vi "select device register.vi"(2 "Camera registers (T) / All Registers (F)":bool, 7 "Ok Button":string) -> (4 "Selected Register":T1, 8 "Register Selected":bool)   [LabVIEW 2010]
panel:
  out "Register Address:":dbl
  out "Raw Register Name:":string
  in  "Cancel":bool
  in  "Select":bool
  out "Pin name on the board:":string
  in  "Register:":u16(ring) items=["Camera on Digital 0 - Bit 0", "Camera on Digital 1 - Bit 0"]
  in  "Device:":u16(ring) items=["Common on all devices", "Behavior", "Camera Controller", "Multi Pwm", "Synchronizer", "Wear"]
  in  "read 5":bool
  in  "read 4":bool
  in  "read":bool
  in  "read 6":bool
  in  "read 7":bool
  in  "read 8":bool
  in  "read 3":bool
  in  "device":refnum<visa-resource-name>="COM5"
  # "Options:"
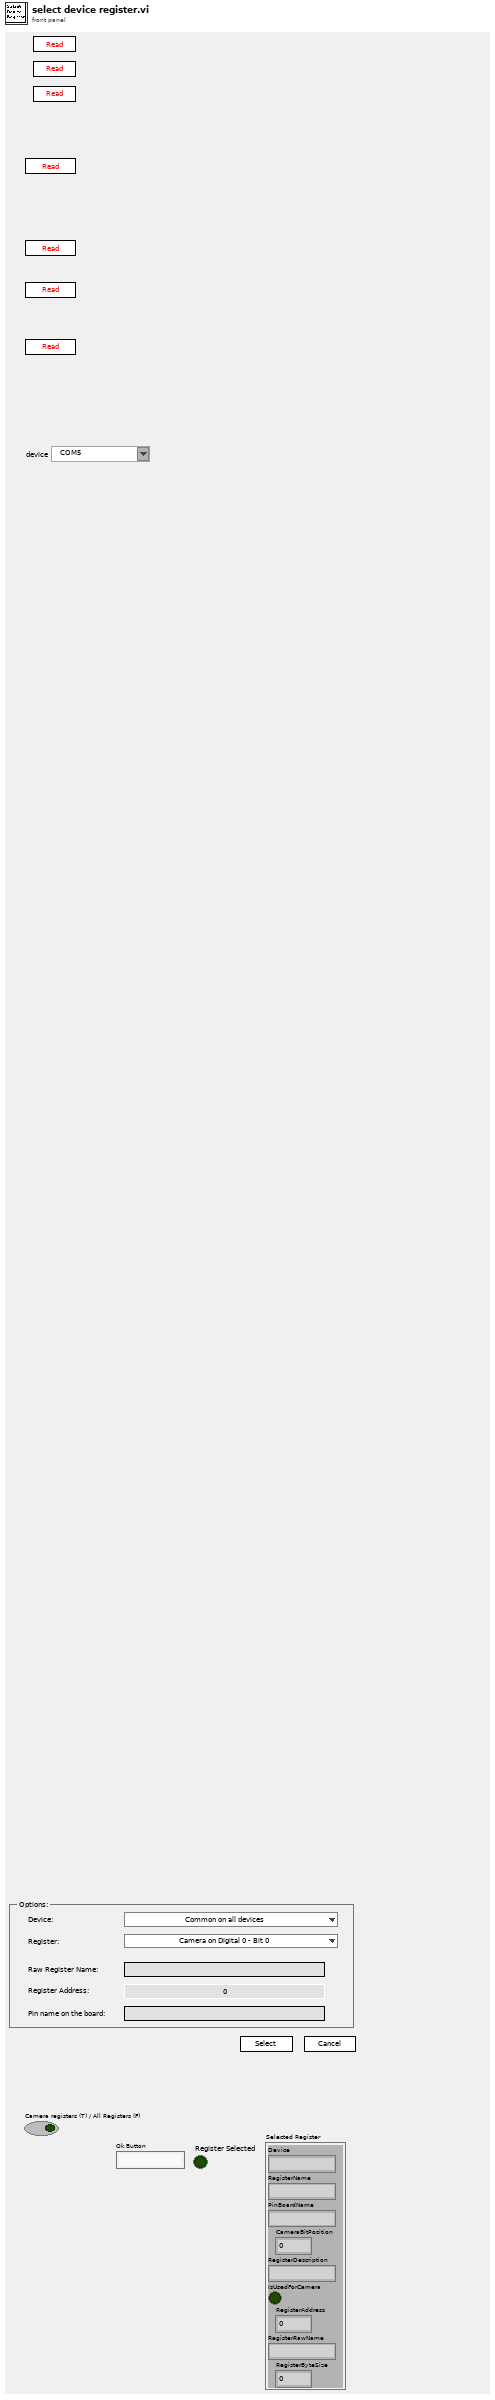
[diagram p1: front panel]
types:
  T1 = cluster{"Device":string, "RegisterName":string, "PinBoardName":string, "CameraBitPosition":i32, "RegisterDescription":string, "IsUsedForCamera":bool, "RegisterAddress":i32, "RegisterRawName":string, "RegisterByteSize":i32}
  T2 = cluster{"Device":string, "RegisterName":string, "PinBoardName":string, "CameraBitPosition":i32, "RegisterDescription":string, "IsUsedForCamera":bool, "RegisterAddress":i32, "RegisterRawName":string, "RegisterByteSize":i32}[][]
  T3 = cluster{"Device":string, "RegisterName":string, "PinBoardName":string, "CameraBitPosition":i32, "RegisterDescription":string, "IsUsedForCamera":bool, "RegisterAddress":i32, "RegisterRawName":string, "RegisterByteSize":i32}[]
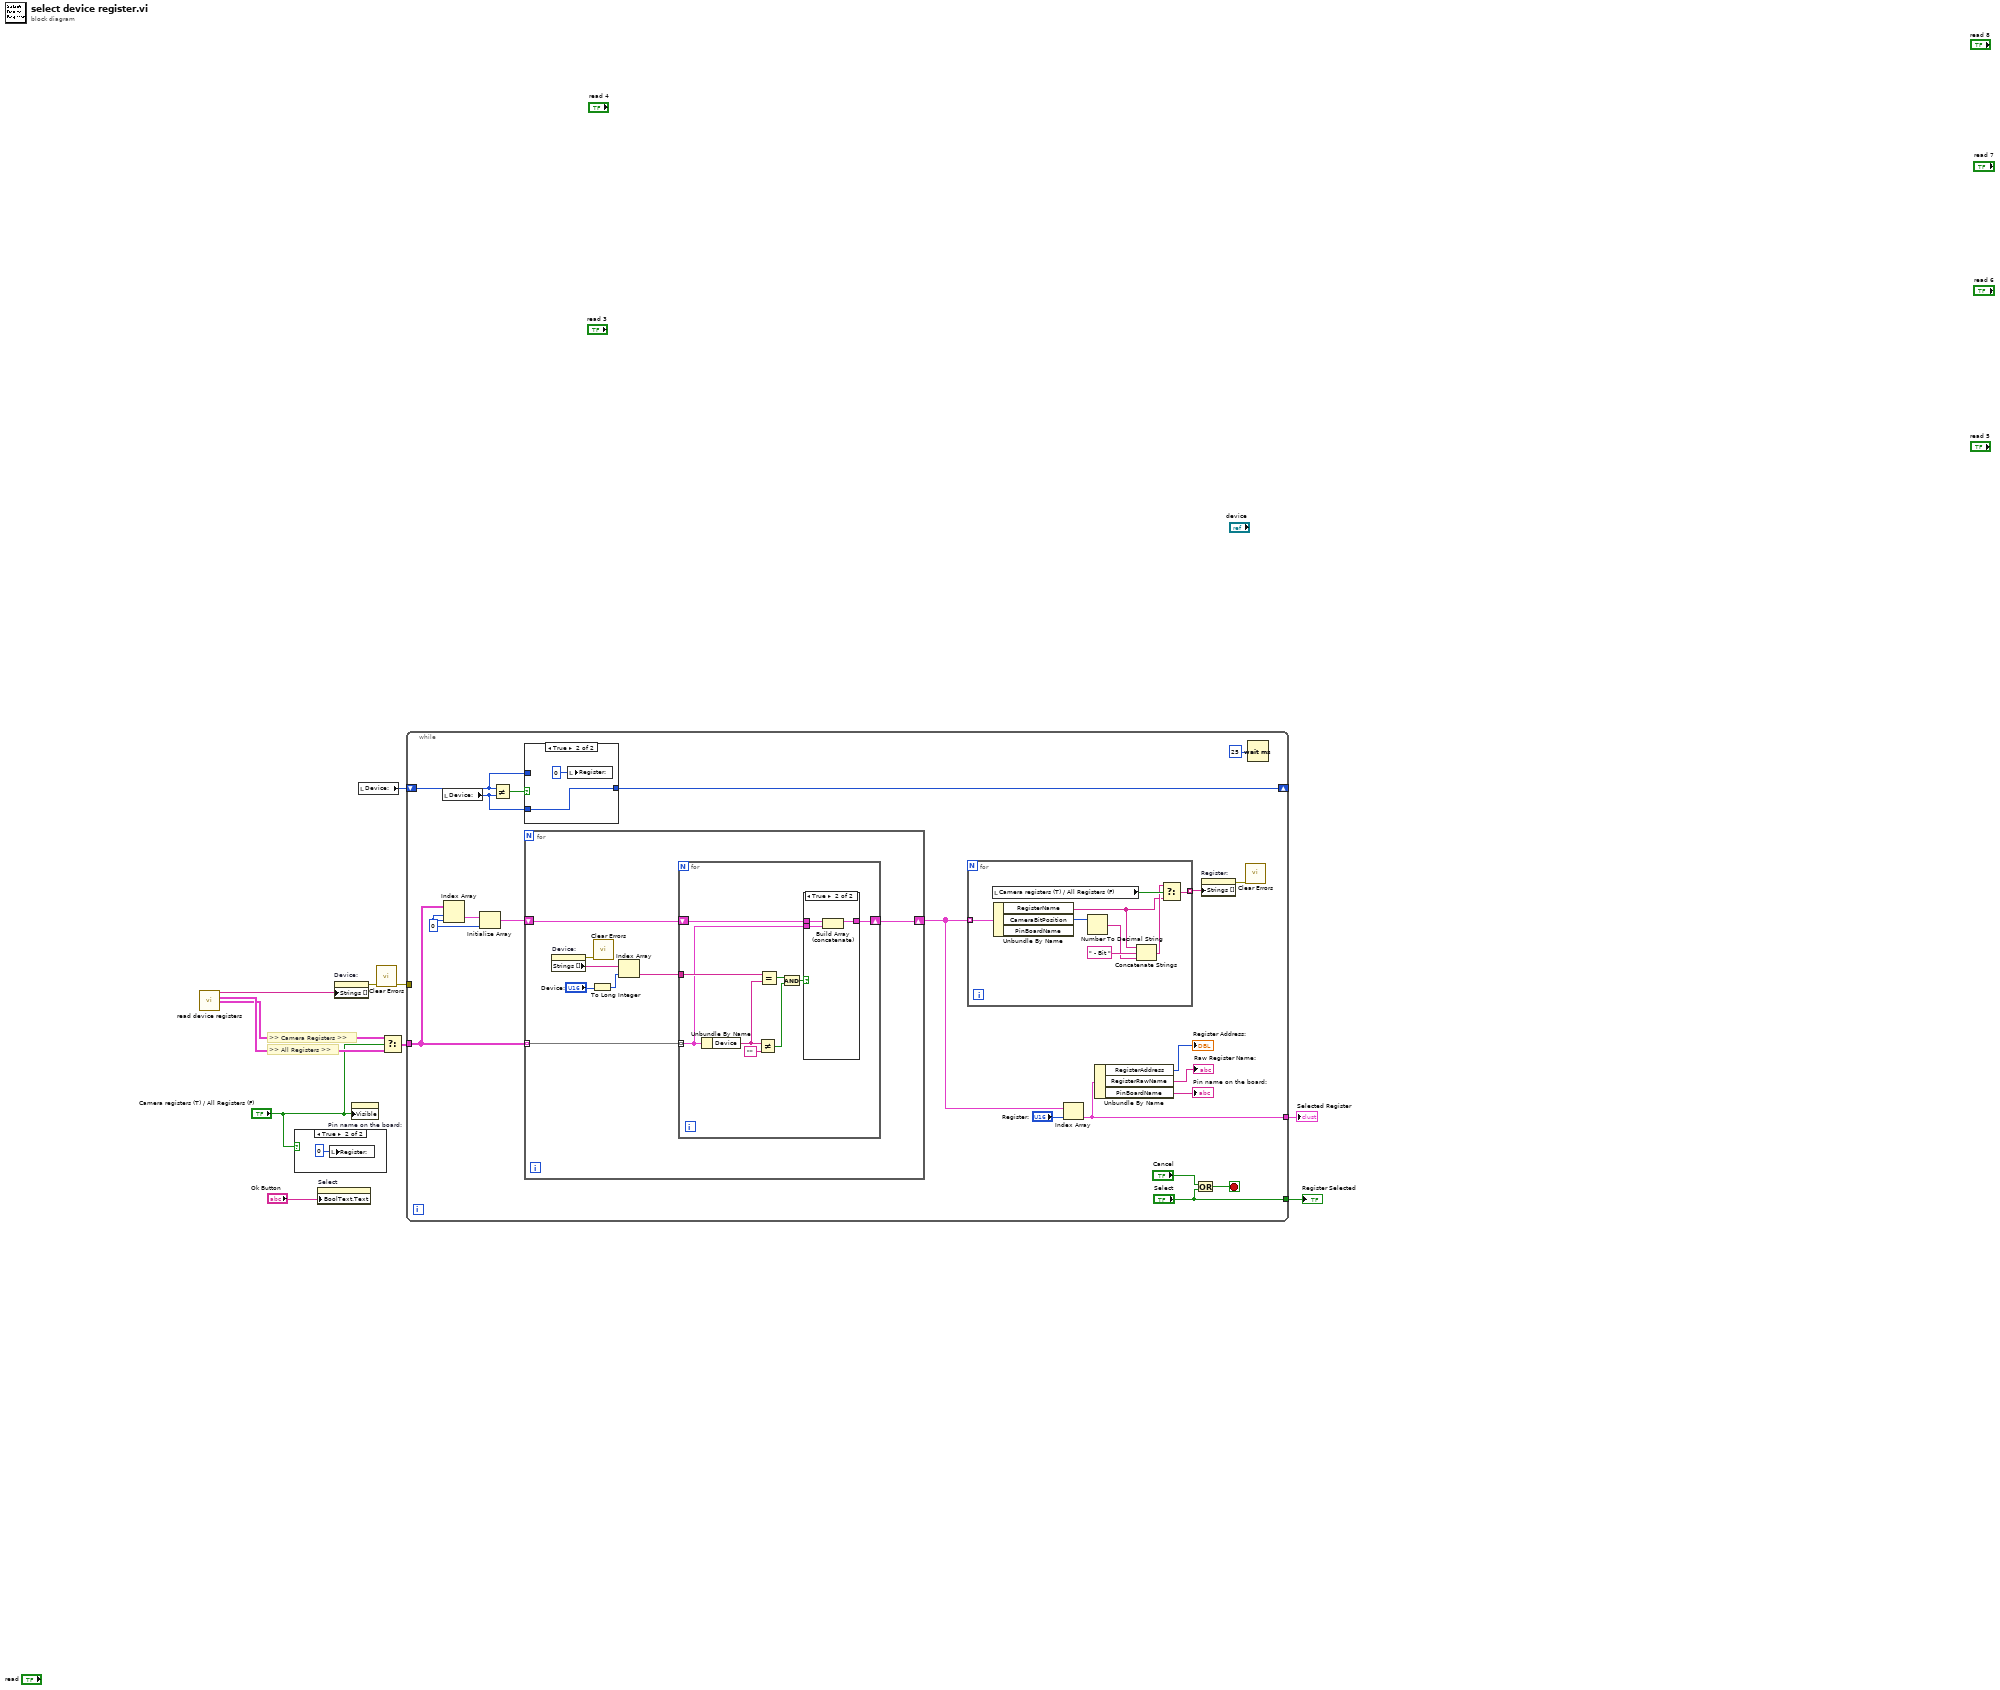
[diagram p0: block diagram]
diagram:
  # ">> Camera Registers >>"
  # ">> All Registers >>"
  n1 = call "read device registers.vi"() -> ("Sorted Device Names"=w6:string[], "All Registers"=w5:T2, "Camera Registers"=w4:T2)  [unwired: 12 in, 1 out]
  n2 = case shown="True" "Camera registers (T) / All Registers (F)" {
    frame False {
    }
    frame True {
      n3 = local write "Register:"(0) -> ()
    }
  }
  n4 = property on="Select" class="Bool"("BoolText.Text"="Ok Button") -> ()  [unwired: 2 in, 2 out]
  n5 = property on="Device:" class="Ring (strict)"("Strings []"=w6) -> (error out=w9:errorcluster)  [unwired: 2 in, 1 out]
  n6 = property on="Pin name on the board:" class="Str"("Visible"="Camera registers (T) / All Registers (F)") -> ()  [unwired: 2 in, 2 out]
  n7 = local read "Device:"() -> (w10:u16)
  n8 = call <vilib>:"Clear Errors.vi"("error in (no error)"=w9) -> ("error out"=w8:errorcluster)  [unwired: 6 in]
  n9 = Select(t=w4, s="Camera registers (T) / All Registers (F)", f=w5) -> (s? t:f=w11:T2)
  n10 = while {
    tunnel: w11 -> [w32]
    shift-right: [w24] -> _
    shift-left: w10 -> [w25]
    tunnel: [w19] -> w2
    tunnel: w8 -> [_]
    tunnel: ["Select"] -> w7
    stop <- w16 stop-if-true
    w30 = 0 ("index (row)")
    n11 = local read "Device:"() -> (w23:u16)
    n12 = Index Array(array=w32, index (row)=w30, index (col)=w30) -> (element=w31:T1)
    n13 = Initialize Array(w31, w30) -> (w29:T3)
    n14 = Not Equal?(x=w25, y=w23) -> (x != y?=w26:bool)
    n15 = for {
      tunnel: w32 -> [w48] mode=indexing
      shift-right: [w46] -> w21
      shift-left: w29 -> [w47]
      n16 = property on="Device:" class="Ring (strict)"() -> (error out=w44:errorcluster, "Strings []"=w50:string[])  [unwired: 2 in, 1 out]
      n17 = To Long Integer(number="Device:") -> (32bit integer=w51:i32)
      n18 = call <vilib>:"Clear Errors.vi"("error in (no error)"=w44) -> ()  [unwired: 6 in, 1 out]
      n19 = Index Array(array=w50, index=w51) -> (element=w49:string)
      n20 = for {
        tunnel: w49 -> [w60]
        tunnel: w48 -> [w52] mode=indexing
        shift-right: [w56] -> w46
        shift-left: w47 -> [w57]
        n21 = Unbundle By Name(w52) -> ("Device"=w59:string)
        n22 = Not Equal?(x=w59, y="") -> (x != y?=w54:bool)
        n23 = Equal?(x=w60, y=w59) -> (x = y?=w55:bool)
        n24 = And(x=w55, y=w54) -> (x .and. y?=w53:bool)
        n25 = case shown="True" w53 {
          tunnel: w57 -> [w61 w64]
          tunnel: [w61 w63] -> w56
          tunnel: w52 -> [_ w62]
          frame False {
          }
          frame True {
            n26 = Build Array (concatenate)(w64, w62) -> (w63:T3)
          }
        }
      }
    }
    n27 = case shown="True" w26 {
      tunnel: w25 -> [w33 _]
      tunnel: [w33 w35] -> w24
      tunnel: w23 -> [_ w35]
      frame False {
      }
      frame True {
        n28 = local write "Register:"(0 ("index (row)")) -> ()
      }
    }
    n29 = for {
      tunnel: w21 -> [w43] mode=indexing
      tunnel: [w36] -> w28 mode=indexing
      n30 = local read "Camera registers (T) / All Registers (F)"() -> (w39:bool)
      n31 = Unbundle By Name(w43) -> ("RegisterName"=w37:string, "CameraBitPosition"=w42:i32)  [unwired: 1 out]
      n32 = Number To Decimal String(number=w42) -> (decimal integer string=w40:string)  [unwired: 1 in]
      n33 = Concatenate Strings(w37, " - Bit " ("string"), w40) -> (w38:string)
      n34 = Select(t=w38, s=w39, f=w37) -> (s? t:f=w36:string)
    }
    n35 = Index Array(array=w21, index="Register:") -> (element=w19:T1)
    n36 = Unbundle By Name(w19) -> ("RegisterAddress"=→"Register Address:":i32, "RegisterRawName"=→"Raw Register Name:":string, "PinBoardName"=→"Pin name on the board:":string)
    n37 = Or(x="Cancel", y="Select") -> (x .or. y?=w16:bool)
    n38 = property on="Register:" class="Ring (strict)"("Strings []"=w28) -> (error out=w27:errorcluster)  [unwired: 2 in, 1 out]
    n39 = call <vilib>:"Clear Errors.vi"("error in (no error)"=w27) -> ()  [unwired: 6 in, 1 out]
    n40 = Wait (ms)(milliseconds to wait=u32 25) -> ()  [unwired: 1 out]
  }
  "Register Selected" <- w7
  "Selected Register" <- w2
